vi "Append.vi"(6 "deadline":T1={"mode"=enum."Relative", "deadline (ms)"=30000}, 8 "error in (no error)":errorcluster, 10 "data":u8[](array[numeric]), 11 "Stream Download Controller in":refnum<class "Stream Download Controller.lvclass">) -> (0 "error out":errorcluster, 3 "Stream Download Controller out":refnum<class "Stream Download Controller.lvclass">)   [LabVIEW 2020, in "NI_SFTP.lvlib" / "Stream Download Controller.lvclass"]
uses:
  <vilib>/net/SFTP/API/Support/Download/Stream/Stream Download Controller.lvclass
  <vilib>/Utility/Deadline/Deadline.ctl
  <vilib>/Utility/Deadline/Mode.ctl
  <vilib>/net/SFTP/API/Support/Download/Stream/Stream Download Controller.lvclass/Stream Download Controller.ctl
  <vilib>/net/SFTP/API/Support/Download/Stream/Element.ctl
  <vilib>/Utility/Deadline/NI_Deadline.lvlib
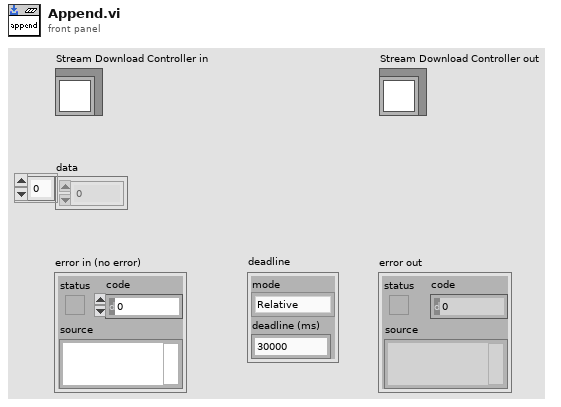
[diagram p1: front panel]
types:
  T1 = typedef "NI_Deadline.lvlib/Deadline.ctl" = cluster{"mode":T2, "deadline (ms)":u32}
  T2 = typedef "NI_Deadline.lvlib/Mode.ctl" = enum16{"Relative", "Use deadline", "Wait forever", "Nonblocking", "N/A"}
  T3 = typedef "NI_SFTP.lvlib/Stream Download Controller.lvclass/Element.ctl" = cluster{"data":u8[], "abort":bool}
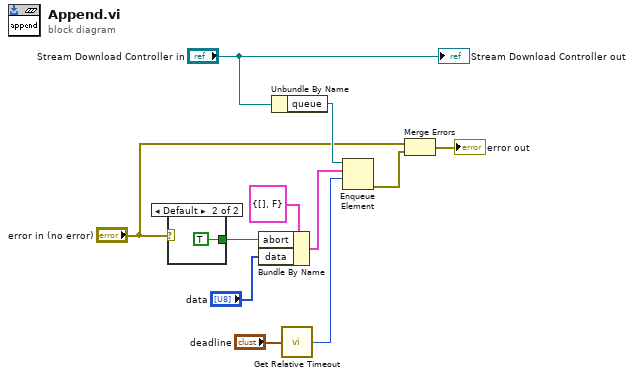
[diagram p0: block diagram]
diagram:
  n1 = case shown="Default" "error in (no error)" {
    tunnel: [_ TRUE] -> w6
    frame No Error {
    }
    frame Default {
    }
  }
  n2 = Bundle By Name(cluster=T3 {"data"=[], "abort"=FALSE} ("element"), "abort"=w6, "data"="data") -> (w4:T3)
  n3 = Unbundle By Name("Stream Download Controller in") -> ("queue"=w9:refnum<queue>)
  n4 = call <vilib>:"Get Relative Timeout.vi"("Timeout"="deadline") -> ("timeout (ms) out"=w8:i32)
  n5 = Enqueue Element(queue=w9, element=w4, timeout in ms (-1)=w8) -> (error out=w2:errorcluster)  [unwired: 1 in, 2 out]
  n6 = Merge Errors("error in (no error)", w2) -> (→"error out":errorcluster)
  "Stream Download Controller out" <- "Stream Download Controller in"
